vi "HP 3325B - Set Sweep (SubVI).vi"(0 "start":ext=1000000.0 format="%.3f", 1 "GPIB Address":string="11", 2 "write?":bool=TRUE, 5 "stop":ext=10000000.0 format="%.3f", 7 "sweep time (s)":ext=10000000.0 format="%.3f", 9 "sweep function (none:0)":u16(ring) items=["no sweep", "linear single", "linear cont.", "log single", "log cont."], 11 "error_in":errorcluster, 12 "write_delay (ms)":u32=20) -> (4 "command string":string, 15 "error out":errorcluster)   [LabVIEW 2022 SP3]
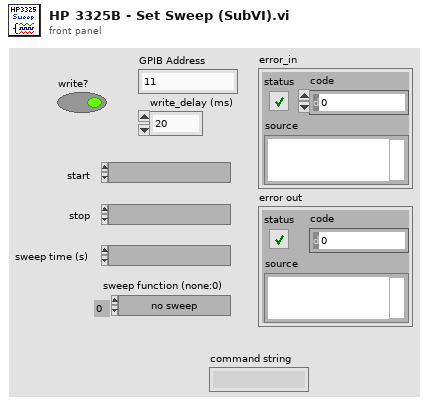
[diagram p1: front panel]
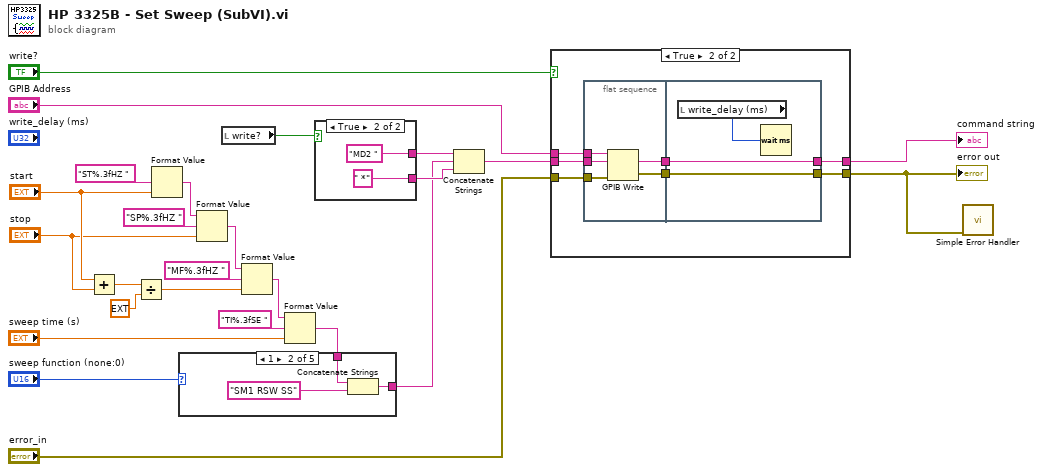
[diagram p0: block diagram]
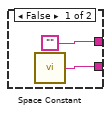
[diagram p2: hidden frame]
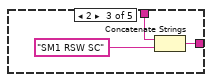
[diagram p4: hidden frame]
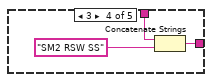
[diagram p5: hidden frame]
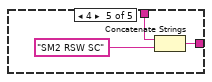
[diagram p6: hidden frame]
diagram:
  n1 = Add(x="start", y="stop") -> (x+y=w19:ext)
  n2 = Divide(x=w19, y=ext 2.0) -> (x/y=w12:ext)
  n3 = Format Value(format string="ST%.3fHZ ", value (0)="start") -> (output string=w13:string)  [unwired: 1 in]
  n4 = Format Value(string ("")=w13, format string="SP%.3fHZ ", value (0)="stop") -> (output string=w11:string)
  n5 = local read "write?"() -> (w5:bool)
  n6 = Format Value(string ("")=w11, format string="MF%.3fHZ ", value (0)=w12) -> (output string=w9:string)
  n7 = Format Value(string ("")=w9, format string="TI%.3fSE ", value (0)="sweep time (s)") -> (output string=w6:string)
  n8 = case shown="1" "sweep function (none:0)" {
    tunnel: w6 -> [w26 w28 w31 w34 w37]
    tunnel: [w26 w29 w32 w35 w38] -> w1
    frame 0, Default {
    }
    frame 1 {
      n9 = Concatenate Strings(w28, "SM1 RSW SS") -> (w29:string)
    }
    frame 2 {
      n10 = Concatenate Strings(w31, "SM1 RSW SC") -> (w32:string)
    }
    frame 3 {
      n11 = Concatenate Strings(w34, "SM2 RSW SS") -> (w35:string)
    }
    frame 4 {
      n12 = Concatenate Strings(w37, "SM2 RSW SC") -> (w38:string)
    }
  }
  n13 = case shown="True" w5 {
    tunnel: [w40 " *"] -> w2
    tunnel: ["" "MD2 " ("string (\"\")")] -> w3
    frame False {
      n14 = call <vilib>:"Space Constant.vi"() -> ("String"=w40:string)
    }
    frame True {
    }
  }
  n15 = Concatenate Strings(w3, w1, w2) -> (w4:string)
  n16 = case shown="True" "write?" {
    tunnel: [w44 w50] -> w24
    tunnel: w4 -> [w43 w49]
    tunnel: "error_in" -> [w44 w48]
    tunnel: "GPIB Address" -> [_ w47]
    tunnel: [w43 w45] -> w20
    frame False {
    }
    frame True {
      n17 = flat-sequence {
        tunnel: w47 -> [w55]
        tunnel: w49 -> [w52]
        tunnel: w48 -> [w53]
        tunnel: [w54] -> w51
        tunnel: [w52] -> w46
        tunnel: [w58] -> w50
        tunnel: w51 -> [w58]
        tunnel: w46 -> [w56]
        tunnel: [w56] -> w45
        frame #0 {
          n18 = GPIB Write(0:w55, 1:w52, 3:w53) -> (6:w54:errorcluster)  [unwired: 2 in, 1 out]
        }
        frame #1 {
          n19 = local read "write_delay (ms)"() -> (w57:u32)
          n20 = Wait (ms)(milliseconds to wait=w57) -> ()  [unwired: 1 out]
        }
      }
    }
  }
  "error out" <- w24
  "command string" <- w20
  n21 = call <vilib>:"Simple Error Handler.vi"("error in (no error)"=w24) -> ()  [unwired: 4 in, 5 out]
